vi "首页.vi"() -> ()   [LabVIEW 2016]
uses:
  <vilib>/Utility/miscctls.llb/LVPointTypeDef.ctl
  API/database/Access/Access Lib.lvlib
panel:
  out "显示":T1
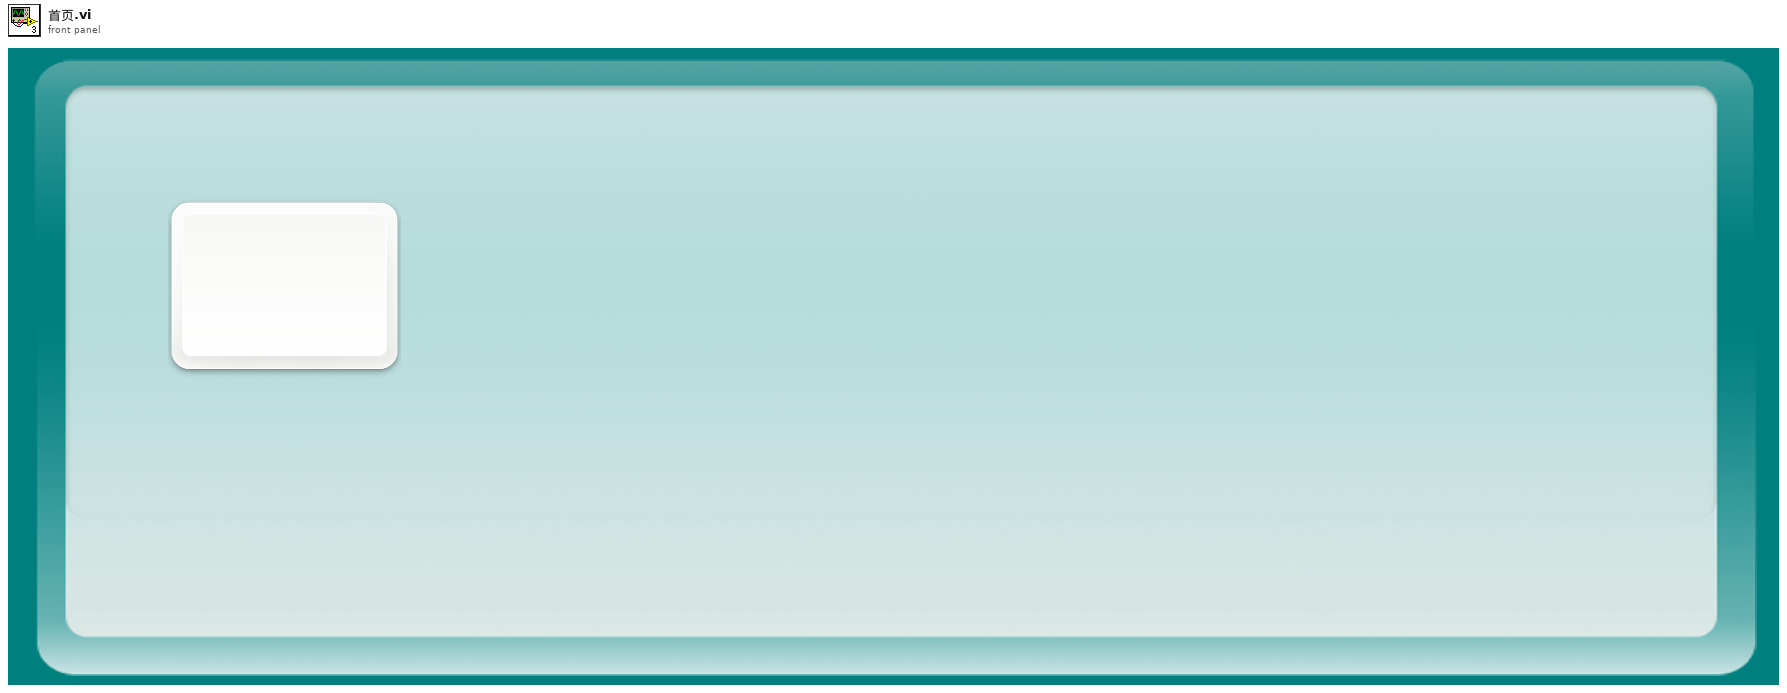
[diagram p1: front panel]
types:
  T1 = typedef "多数值显示.ctl" = cluster{"显示":T2, "显示 2":T2, "显示 3":T2, "显示 4":T2, "显示 5":T2, "显示 6":T2, "显示 12":T2, "显示 11":T2, "显示 10":T2, "显示 9":T2, "显示 8":T2, "显示 7":T2}
  T2 = typedef "数值显示.ctl" = cluster{"中文项目名称":string, "英文项目名称":string, "浓度":string, "单位":string}
  T3 = typedef "LVPointTypeDef.ctl" = cluster{"Horizontal":i16, "Vertical":i16}
  T4 = cluster{"显示参数中文名":string, "显示参数英文名":string, "显示浓度":string, "显示单位":string}[]
  T5 = cluster{"显示参数中文名":string, "显示参数英文名":string, "显示浓度":string, "显示单位":string}
  T6 = cluster{"水温":bool, "pH":bool, "DO":bool, "Cond":bool, "Turb":bool, "氨氮":bool, "总磷":bool, "总氮":bool, "CODMn":bool, "CODCr":bool, "水位":bool, "流速":bool, "瞬时流量":bool, "ORP":bool, "氟化物":bool, "铅":bool, "镉":bool, "铜":bool, "锌":bool, "汞":bool, "叶绿素a":bool, "藻密度":bool, "氯化物":bool, "挥发酚":bool, "盐度":bool}
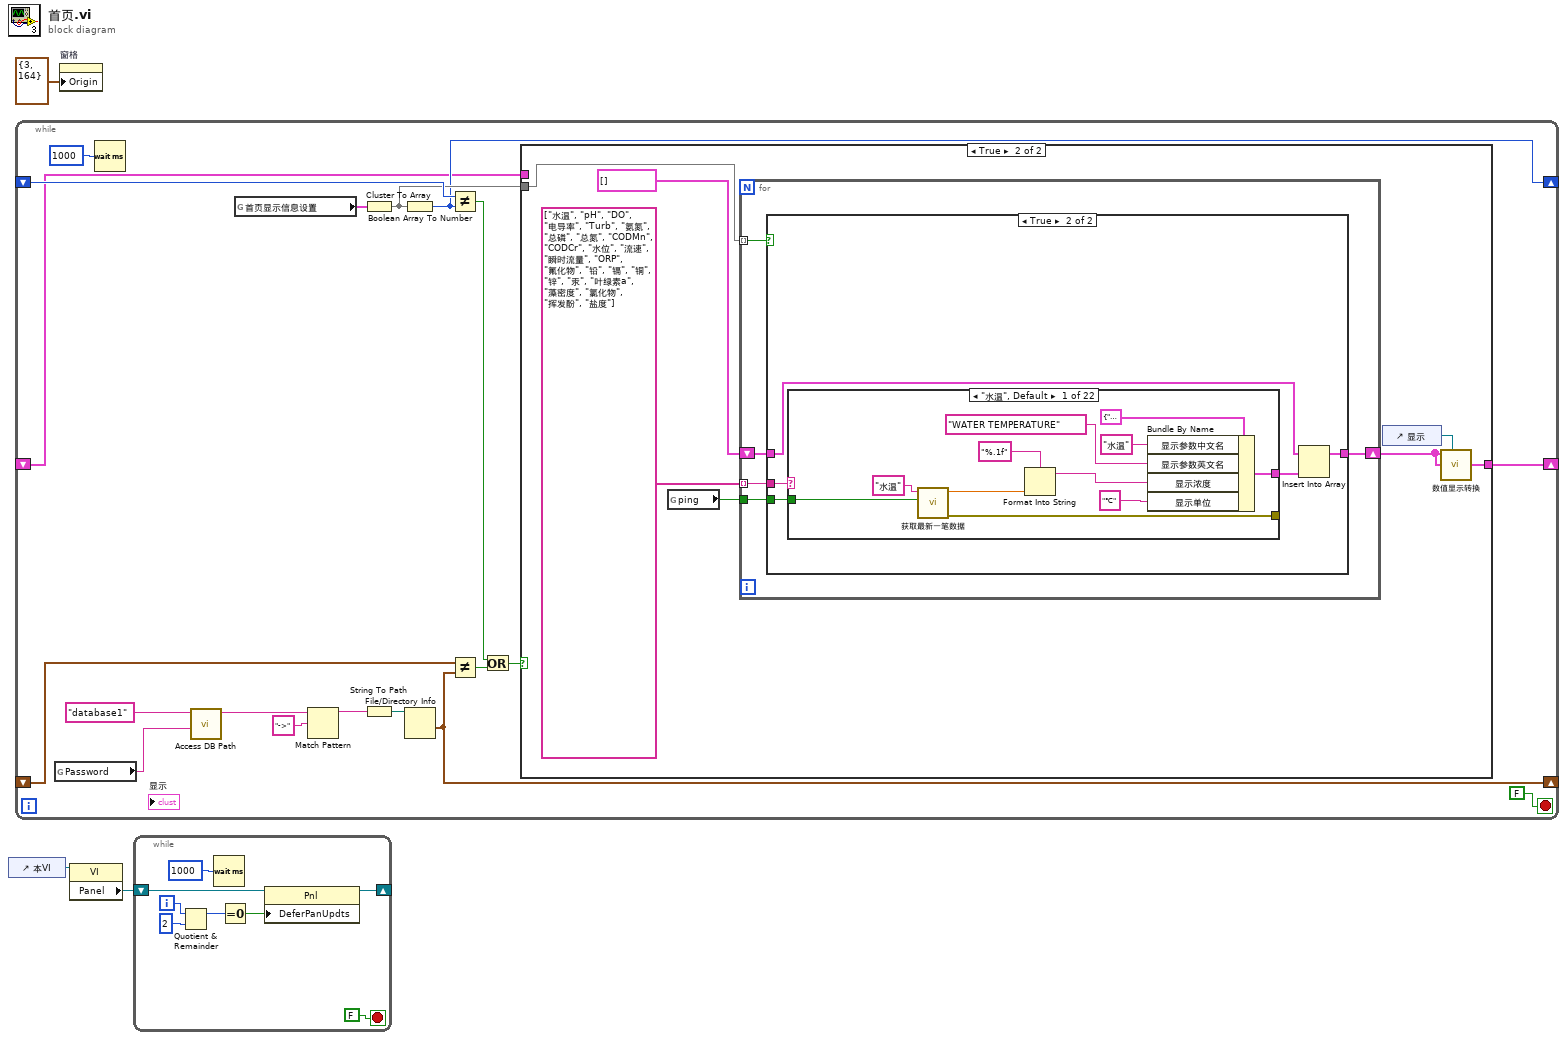
[diagram p0: block diagram]
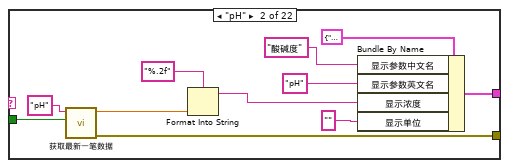
[diagram p4: hidden frame]
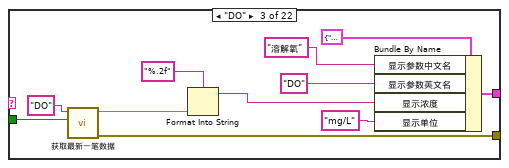
[diagram p5: hidden frame]
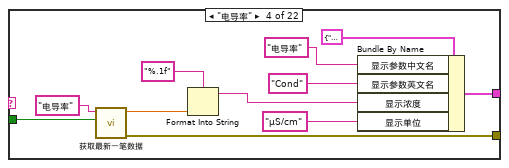
[diagram p6: hidden frame]
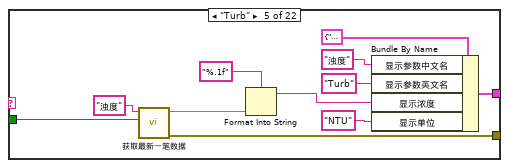
[diagram p7: hidden frame]
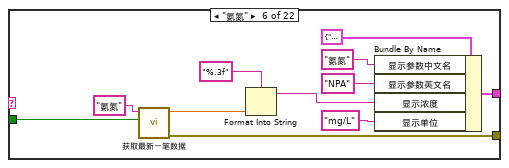
[diagram p8: hidden frame]
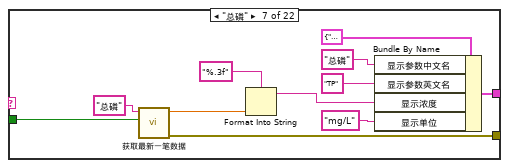
[diagram p9: hidden frame]
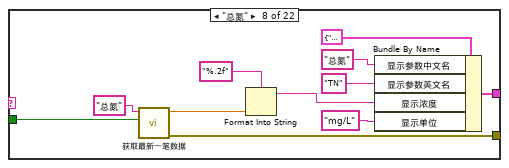
[diagram p10: hidden frame]
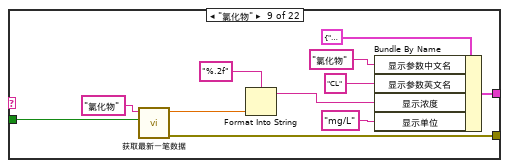
[diagram p11: hidden frame]
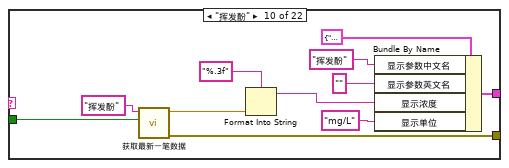
[diagram p12: hidden frame]
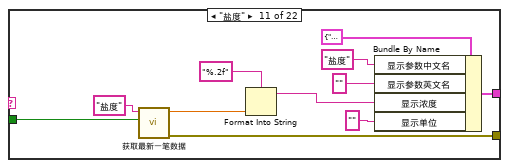
[diagram p13: hidden frame]
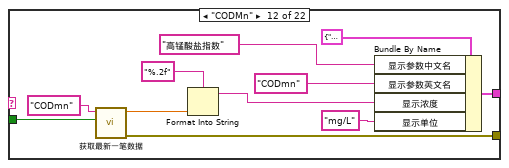
[diagram p14: hidden frame]
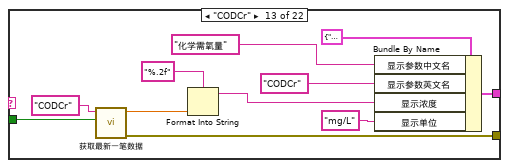
[diagram p15: hidden frame]
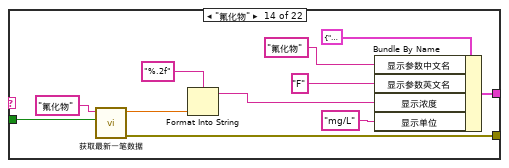
[diagram p16: hidden frame]
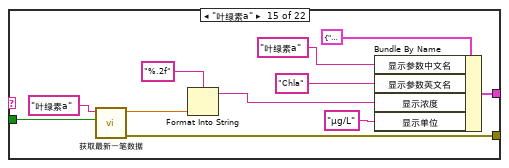
[diagram p17: hidden frame]
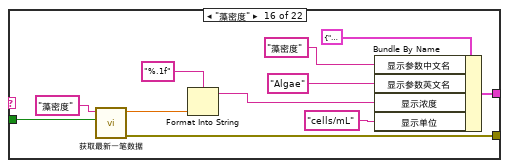
[diagram p18: hidden frame]
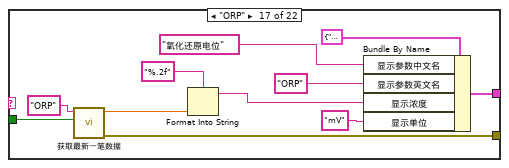
[diagram p19: hidden frame]
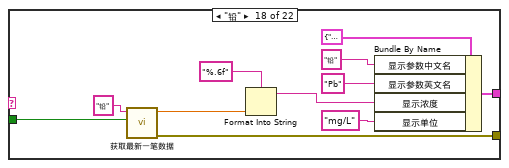
[diagram p20: hidden frame]
diagram:
  n1 = control-ref of="本VI"() -> (w2:refnum<vi>)
  n2 = while {
    shift-right: [w17] -> _
    shift-left: _ -> [w19]
    shift-right: [w5] -> _
    shift-left: _ -> [w16]
    shift-right: [w6] -> _
    shift-left: _ -> [w12]
    stop <- FALSE stop-if-true
    n3 = global read "非断电保持全局变量.vi" "Password"() -> (w4:string)
    n4 = Wait (ms)(milliseconds to wait=u32 1000 ("等待时间（毫秒）")) -> ()  [unwired: 1 out]
    n5 = call "Access DB Path.vi"("Password"=w4, "database"="database1") -> ("Path out"=w10:string)  [unwired: 8 in, 1 out]
    n6 = global read "系统设置全局变量.vi" "首页显示信息设置"() -> (w20:T6)
    n7 = Match Pattern(string=w10, regular expression="->" ("正则表达式")) -> (before substring=w8:string)  [unwired: 1 in, 3 out]
    n8 = Cluster To Array(cluster=w20) -> (array=w18:bool[])
    n9 = String To Path(string=w8) -> (path=w7:path)
    n10 = Boolean Array To Number(Boolean array=w18) -> (number=w17:u32)
    n11 = File/Directory Info(path=w7) -> (last mod=w5:timestamp)  [unwired: 1 in, 6 out]
    n12 = Not Equal?(x=w19, y=w17) -> (x != y?=w13:bool)
    n13 = Not Equal?(x=w16, y=w5) -> (x != y?=w15:bool)
    n14 = Or(x=w13, y=w15) -> (x .or. y?=w14:bool)
    n15 = case shown="True" w14 {
      tunnel: w18 -> [_ w27]
      tunnel: [w23 w24] -> w6
      tunnel: w12 -> [w23 _]
      frame False {
      }
      frame True {
        n16 = global read "全局变量.vi" "ping"() -> (w26:bool)
        n17 = for {
          tunnel: w27 -> [w34] mode=indexing
          tunnel: string[] ["水温", "pH", "DO", "电导率", "Turb", "氨氮", "总磷", "总氮", "CODMn", "CODCr", "水位", "流速", "瞬时流量", "ORP", "氟化物", "铅", "镉", "铜", "锌", "汞", "叶绿素a", "藻密度", "氯化物", "挥发酚", "盐度"] -> [w33] mode=indexing
          shift-right: [w31] -> w24
          shift-left: T4 [] -> [w32]
          tunnel: w26 -> [w30]
          n18 = case shown="True" w34 {
            tunnel: w33 -> [_ w40]
            tunnel: w32 -> [w35 w39]
            tunnel: [w35 w38] -> w31
            tunnel: w30 -> [_ w36]
            frame False {
            }
            frame True {
              n19 = case shown="\"水温\", Default" w40 {
                selector: w40 -> [_ _ _ _ _ _ _ _ _ _ _ _ _ _ _ _ _ _ w239 w249 w259 w269]
                tunnel: [w44 w58 w69 w80 w91 w102 w113 w124 w135 w146 w157 w168 w179 w190 w201 w212 w223 w234 w245 w255 w265 w275] -> w37
                tunnel: [w45 w55 w66 w77 w88 w99 w110 w121 w132 w143 w154 w165 w176 w187 w198 w209 w220 w231 w242 w252 w262 w272] -> _
                tunnel: w36 -> [w41 w52 w63 w74 w85 w96 w107 w118 w129 w140 w151 w162 w173 w184 w195 w206 w217 w228 w240 w250 w260 w270]
                frame "水温", Default {
                  n20 = call "获取最新一笔数据.vi"("ping"=w41, "table"="水温") -> ("错误输出"=w45:errorcluster, "data"=w42:dbl)  [unwired: 7 in, 1 out]
                  n21 = Format Into String(format string="%.1f" ("格式字符串"), w42) -> (resulting string=w46:string)  [unwired: 2 in, 1 out]
                  n22 = Bundle By Name(cluster=T5 {"显示参数中文名"="", "显示参数英文名"="", "显示浓度"="", "显示单位"=""} ("元素"), "显示参数中文名"="水温", "显示参数英文名"="WATER TEMPERATURE", "显示浓度"=w46, "显示单位"="℃") -> (w44:T5)
                }
                frame "pH" {
                  n23 = call "获取最新一笔数据.vi"("ping"=w52, "table"="pH") -> ("错误输出"=w55:errorcluster, "data"=w53:dbl)  [unwired: 7 in, 1 out]
                  n24 = Format Into String(format string="%.2f" ("格式字符串"), w53) -> (resulting string=w56:string)  [unwired: 2 in, 1 out]
                  n25 = Bundle By Name(cluster=T5 {"显示参数中文名"="", "显示参数英文名"="", "显示浓度"="", "显示单位"=""} ("元素"), "显示参数中文名"="酸碱度", "显示参数英文名"="pH", "显示浓度"=w56, "显示单位"="") -> (w58:T5)
                }
                frame "DO" {
                  n26 = call "获取最新一笔数据.vi"("ping"=w63, "table"="DO") -> ("错误输出"=w66:errorcluster, "data"=w64:dbl)  [unwired: 7 in, 1 out]
                  n27 = Format Into String(format string="%.2f" ("格式字符串"), w64) -> (resulting string=w67:string)  [unwired: 2 in, 1 out]
                  n28 = Bundle By Name(cluster=T5 {"显示参数中文名"="", "显示参数英文名"="", "显示浓度"="", "显示单位"=""} ("元素"), "显示参数中文名"="溶解氧", "显示参数英文名"="DO", "显示浓度"=w67, "显示单位"="mg/L") -> (w69:T5)
                }
                frame "电导率" {
                  n29 = call "获取最新一笔数据.vi"("ping"=w74, "table"="电导率") -> ("错误输出"=w77:errorcluster, "data"=w75:dbl)  [unwired: 7 in, 1 out]
                  n30 = Format Into String(format string="%.1f" ("格式字符串"), w75) -> (resulting string=w78:string)  [unwired: 2 in, 1 out]
                  n31 = Bundle By Name(cluster=T5 {"显示参数中文名"="", "显示参数英文名"="", "显示浓度"="", "显示单位"=""} ("元素"), "显示参数中文名"="电导率", "显示参数英文名"="Cond", "显示浓度"=w78, "显示单位"="μS/cm") -> (w80:T5)
                }
                frame "Turb" {
                  n32 = call "获取最新一笔数据.vi"("ping"=w85, "table"="浊度") -> ("错误输出"=w88:errorcluster, "data"=w86:dbl)  [unwired: 7 in, 1 out]
                  n33 = Format Into String(format string="%.1f" ("格式字符串"), w86) -> (resulting string=w89:string)  [unwired: 2 in, 1 out]
                  n34 = Bundle By Name(cluster=T5 {"显示参数中文名"="", "显示参数英文名"="", "显示浓度"="", "显示单位"=""} ("元素"), "显示参数中文名"="浊度", "显示参数英文名"="Turb", "显示浓度"=w89, "显示单位"="NTU") -> (w91:T5)
                }
                frame "氨氮" {
                  n35 = call "获取最新一笔数据.vi"("ping"=w96, "table"="氨氮") -> ("错误输出"=w99:errorcluster, "data"=w98:dbl)  [unwired: 7 in, 1 out]
                  n36 = Format Into String(format string="%.3f" ("格式字符串"), w98) -> (resulting string=w100:string)  [unwired: 2 in, 1 out]
                  n37 = Bundle By Name(cluster=T5 {"显示参数中文名"="", "显示参数英文名"="", "显示浓度"="", "显示单位"=""} ("元素"), "显示参数中文名"="氨氮", "显示参数英文名"="NPA", "显示浓度"=w100, "显示单位"="mg/L") -> (w102:T5)
                }
                frame "总磷" {
                  n38 = call "获取最新一笔数据.vi"("ping"=w107, "table"="总磷") -> ("错误输出"=w110:errorcluster, "data"=w109:dbl)  [unwired: 7 in, 1 out]
                  n39 = Format Into String(format string="%.3f" ("格式字符串"), w109) -> (resulting string=w111:string)  [unwired: 2 in, 1 out]
                  n40 = Bundle By Name(cluster=T5 {"显示参数中文名"="", "显示参数英文名"="", "显示浓度"="", "显示单位"=""} ("元素"), "显示参数中文名"="总磷", "显示参数英文名"="TP", "显示浓度"=w111, "显示单位"="mg/L") -> (w113:T5)
                }
                frame "总氮" {
                  n41 = call "获取最新一笔数据.vi"("ping"=w118, "table"="总氮") -> ("错误输出"=w121:errorcluster, "data"=w120:dbl)  [unwired: 7 in, 1 out]
                  n42 = Format Into String(format string="%.2f" ("格式字符串"), w120) -> (resulting string=w122:string)  [unwired: 2 in, 1 out]
                  n43 = Bundle By Name(cluster=T5 {"显示参数中文名"="", "显示参数英文名"="", "显示浓度"="", "显示单位"=""} ("元素"), "显示参数中文名"="总氮", "显示参数英文名"="TN", "显示浓度"=w122, "显示单位"="mg/L") -> (w124:T5)
                }
                frame "氯化物" {
                  n44 = call "获取最新一笔数据.vi"("ping"=w129, "table"="氯化物") -> ("错误输出"=w132:errorcluster, "data"=w131:dbl)  [unwired: 7 in, 1 out]
                  n45 = Format Into String(format string="%.2f" ("格式字符串"), w131) -> (resulting string=w133:string)  [unwired: 2 in, 1 out]
                  n46 = Bundle By Name(cluster=T5 {"显示参数中文名"="", "显示参数英文名"="", "显示浓度"="", "显示单位"=""} ("元素"), "显示参数中文名"="氯化物", "显示参数英文名"="CL", "显示浓度"=w133, "显示单位"="mg/L") -> (w135:T5)
                }
                frame "挥发酚" {
                  n47 = call "获取最新一笔数据.vi"("ping"=w140, "table"="挥发酚") -> ("错误输出"=w143:errorcluster, "data"=w142:dbl)  [unwired: 7 in, 1 out]
                  n48 = Format Into String(format string="%.3f" ("格式字符串"), w142) -> (resulting string=w144:string)  [unwired: 2 in, 1 out]
                  n49 = Bundle By Name(cluster=T5 {"显示参数中文名"="", "显示参数英文名"="", "显示浓度"="", "显示单位"=""} ("元素"), "显示参数中文名"="挥发酚", "显示参数英文名"="", "显示浓度"=w144, "显示单位"="mg/L") -> (w146:T5)
                }
                frame "盐度" {
                  n50 = call "获取最新一笔数据.vi"("ping"=w151, "table"="盐度") -> ("错误输出"=w154:errorcluster, "data"=w153:dbl)  [unwired: 7 in, 1 out]
                  n51 = Format Into String(format string="%.2f" ("格式字符串"), w153) -> (resulting string=w155:string)  [unwired: 2 in, 1 out]
                  n52 = Bundle By Name(cluster=T5 {"显示参数中文名"="", "显示参数英文名"="", "显示浓度"="", "显示单位"=""} ("元素"), "显示参数中文名"="盐度", "显示参数英文名"="", "显示浓度"=w155, "显示单位"="") -> (w157:T5)
                }
                frame "CODMn" {
                  n53 = call "获取最新一笔数据.vi"("ping"=w162, "table"="CODmn") -> ("错误输出"=w165:errorcluster, "data"=w164:dbl)  [unwired: 7 in, 1 out]
                  n54 = Format Into String(format string="%.2f" ("格式字符串"), w164) -> (resulting string=w166:string)  [unwired: 2 in, 1 out]
                  n55 = Bundle By Name(cluster=T5 {"显示参数中文名"="", "显示参数英文名"="", "显示浓度"="", "显示单位"=""} ("元素"), "显示参数中文名"="高锰酸盐指数", "显示参数英文名"="CODmn", "显示浓度"=w166, "显示单位"="mg/L") -> (w168:T5)
                }
                frame "CODCr" {
                  n56 = call "获取最新一笔数据.vi"("ping"=w173, "table"="CODCr") -> ("错误输出"=w176:errorcluster, "data"=w175:dbl)  [unwired: 7 in, 1 out]
                  n57 = Format Into String(format string="%.2f" ("格式字符串"), w175) -> (resulting string=w177:string)  [unwired: 2 in, 1 out]
                  n58 = Bundle By Name(cluster=T5 {"显示参数中文名"="", "显示参数英文名"="", "显示浓度"="", "显示单位"=""} ("元素"), "显示参数中文名"="化学需氧量", "显示参数英文名"="CODCr", "显示浓度"=w177, "显示单位"="mg/L") -> (w179:T5)
                }
                frame "氟化物" {
                  n59 = call "获取最新一笔数据.vi"("ping"=w184, "table"="氟化物") -> ("错误输出"=w187:errorcluster, "data"=w186:dbl)  [unwired: 7 in, 1 out]
                  n60 = Format Into String(format string="%.2f" ("格式字符串"), w186) -> (resulting string=w188:string)  [unwired: 2 in, 1 out]
                  n61 = Bundle By Name(cluster=T5 {"显示参数中文名"="", "显示参数英文名"="", "显示浓度"="", "显示单位"=""} ("元素"), "显示参数中文名"="氟化物", "显示参数英文名"="F", "显示浓度"=w188, "显示单位"="mg/L") -> (w190:T5)
                }
                frame "叶绿素a" {
                  n62 = call "获取最新一笔数据.vi"("ping"=w195, "table"="叶绿素a") -> ("错误输出"=w198:errorcluster, "data"=w197:dbl)  [unwired: 7 in, 1 out]
                  n63 = Format Into String(format string="%.2f" ("格式字符串"), w197) -> (resulting string=w199:string)  [unwired: 2 in, 1 out]
                  n64 = Bundle By Name(cluster=T5 {"显示参数中文名"="", "显示参数英文名"="", "显示浓度"="", "显示单位"=""} ("元素"), "显示参数中文名"="叶绿素a", "显示参数英文名"="Chla", "显示浓度"=w199, "显示单位"="μg/L") -> (w201:T5)
                }
                frame "藻密度" {
                  n65 = call "获取最新一笔数据.vi"("ping"=w206, "table"="藻密度") -> ("错误输出"=w209:errorcluster, "data"=w208:dbl)  [unwired: 7 in, 1 out]
                  n66 = Format Into String(format string="%.1f" ("格式字符串"), w208) -> (resulting string=w210:string)  [unwired: 2 in, 1 out]
                  n67 = Bundle By Name(cluster=T5 {"显示参数中文名"="", "显示参数英文名"="", "显示浓度"="", "显示单位"=""} ("元素"), "显示参数中文名"="藻密度", "显示参数英文名"="Algae", "显示浓度"=w210, "显示单位"="cells/mL") -> (w212:T5)
                }
                frame "ORP" {
                  n68 = call "获取最新一笔数据.vi"("ping"=w217, "table"="ORP") -> ("错误输出"=w220:errorcluster, "data"=w219:dbl)  [unwired: 7 in, 1 out]
                  n69 = Format Into String(format string="%.2f" ("格式字符串"), w219) -> (resulting string=w221:string)  [unwired: 2 in, 1 out]
                  n70 = Bundle By Name(cluster=T5 {"显示参数中文名"="", "显示参数英文名"="", "显示浓度"="", "显示单位"=""} ("元素"), "显示参数中文名"="氧化还原电位", "显示参数英文名"="ORP", "显示浓度"=w221, "显示单位"="mV") -> (w223:T5)
                }
                frame "铅" {
                  n71 = call "获取最新一笔数据.vi"("ping"=w228, "table"="铅") -> ("错误输出"=w231:errorcluster, "data"=w230:dbl)  [unwired: 7 in, 1 out]
                  n72 = Format Into String(format string="%.6f" ("格式字符串"), w230) -> (resulting string=w232:string)  [unwired: 2 in, 1 out]
                  n73 = Bundle By Name(cluster=T5 {"显示参数中文名"="", "显示参数英文名"="", "显示浓度"="", "显示单位"=""} ("元素"), "显示参数中文名"="铅", "显示参数英文名"="Pb", "显示浓度"=w232, "显示单位"="mg/L") -> (w234:T5)
                }
                frame "镉" {
                  n74 = call "获取最新一笔数据.vi"("ping"=w240, "table"=w239) -> ("错误输出"=w242:errorcluster, "data"=w241:dbl)  [unwired: 7 in, 1 out]
                  n75 = Format Into String(format string="%.6f" ("格式字符串"), w241) -> (resulting string=w243:string)  [unwired: 2 in, 1 out]
                  n76 = Bundle By Name(cluster=T5 {"显示参数中文名"="", "显示参数英文名"="", "显示浓度"="", "显示单位"=""} ("元素"), "显示参数中文名"=w239, "显示参数英文名"="Cd", "显示浓度"=w243, "显示单位"="mg/L") -> (w245:T5)
                }
                frame "铜" {
                  n77 = call "获取最新一笔数据.vi"("ping"=w250, "table"=w249) -> ("错误输出"=w252:errorcluster, "data"=w251:dbl)  [unwired: 7 in, 1 out]
                  n78 = Format Into String(format string="%.6f" ("格式字符串"), w251) -> (resulting string=w253:string)  [unwired: 2 in, 1 out]
                  n79 = Bundle By Name(cluster=T5 {"显示参数中文名"="", "显示参数英文名"="", "显示浓度"="", "显示单位"=""} ("元素"), "显示参数中文名"=w249, "显示参数英文名"="Cu", "显示浓度"=w253, "显示单位"="mg/L") -> (w255:T5)
                }
                frame "锌" {
                  n80 = call "获取最新一笔数据.vi"("ping"=w260, "table"=w259) -> ("错误输出"=w262:errorcluster, "data"=w261:dbl)  [unwired: 7 in, 1 out]
                  n81 = Format Into String(format string="%.6f" ("格式字符串"), w261) -> (resulting string=w263:string)  [unwired: 2 in, 1 out]
                  n82 = Bundle By Name(cluster=T5 {"显示参数中文名"="", "显示参数英文名"="", "显示浓度"="", "显示单位"=""} ("元素"), "显示参数中文名"=w259, "显示参数英文名"="Zn", "显示浓度"=w263, "显示单位"="mg/L") -> (w265:T5)
                }
                frame "总汞" {
                  n83 = call "获取最新一笔数据.vi"("ping"=w270, "table"=w269) -> ("错误输出"=w272:errorcluster, "data"=w271:dbl)  [unwired: 7 in, 1 out]
                  n84 = Format Into String(format string="%.6f" ("格式字符串"), w271) -> (resulting string=w273:string)  [unwired: 2 in, 1 out]
                  n85 = Bundle By Name(cluster=T5 {"显示参数中文名"="", "显示参数英文名"="", "显示浓度"="", "显示单位"=""} ("元素"), "显示参数中文名"=w269, "显示参数英文名"="Hg", "显示浓度"=w273, "显示单位"="mg/L") -> (w275:T5)
                }
              }
              n86 = Insert Into Array(array=w39, new element=w37) -> (w38:T4)  [unwired: 1 in]
            }
          }
        }
        n87 = control-ref of="显示"() -> (w25:refnum<vi>)
        n88 = call "数值显示转换.vi"("显示"=w25, "数组"=w24) -> ()  [unwired: 10 in]
      }
    }
  }
  n89 = property on="窗格" class="Pane"("Origin"=T3 {"Horizontal"=3, "Vertical"=164} ("原点")) -> ()  [unwired: 2 in, 2 out]
  n90 = property class="VI"(reference=w2) -> ("Panel"=w1:refnum<vi>)  [unwired: 1 in, 2 out]
  n91 = while {
    shift-right: [w279] -> _
    shift-left: w1 -> [w284]
    i -> [w283]
    stop <- FALSE stop-if-true
    n92 = Quotient & Remainder(x=w283, y=2) -> (x-y*floor(x/y)=w281:i32)  [unwired: 1 out]
    n93 = Wait (ms)(milliseconds to wait=u32 1000 ("等待时间（毫秒）")) -> ()  [unwired: 1 out]
    n94 = Equal To 0?(x=w281) -> (x = 0?=w280:bool)
    n95 = property class="Pnl"(reference=w284, "DeferPanUpdts"=w280) -> (reference out=w279:refnum<vi>)  [unwired: 1 in, 1 out]
  }
